vi "Get Names.vi"(8 "error in (no error)":errorcluster, 11 "Red Plugin in":refnum<class "Red Plugin.lvclass">) -> (0 "error out":errorcluster, 2 "Name":string, 3 "Red Plugin out":refnum<class "Red Plugin.lvclass">)   [LabVIEW 2020, in "Red Plugin.lvclass"]
uses:
  Red Plugin.lvclass
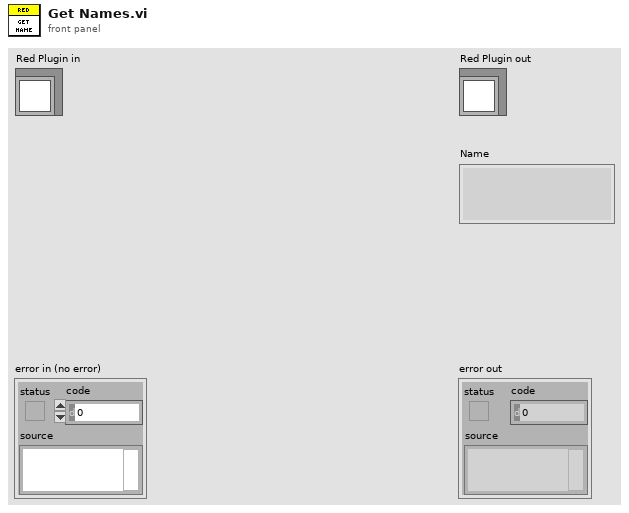
[diagram p1: front panel]
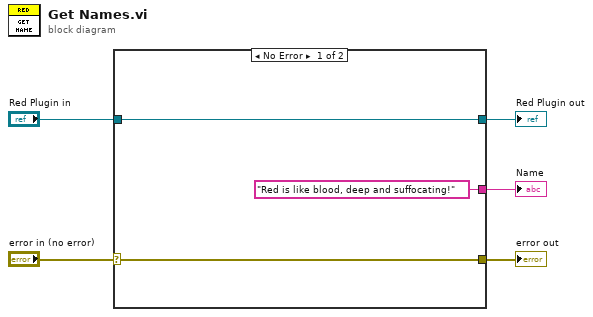
[diagram p0: block diagram]
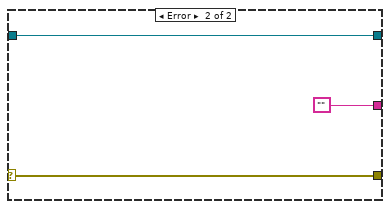
[diagram p2: hidden frame]
diagram:
  n1 = case shown="No Error" "error in (no error)" {
    selector: "error in (no error)" -> [w8 w11]
    tunnel: [w8 w11] -> w4
    tunnel: "Red Plugin in" -> [w7 w10]
    tunnel: [w7 w10] -> w2
    tunnel: ["Red is like blood, deep and suffocating!" ""] -> w1
    frame No Error {
    }
    frame Error {
    }
  }
  "error out" <- w4
  "Red Plugin out" <- w2
  "Name" <- w1
